vi "Message type that caused error.vi"(11 "ErrorHandler MsgPack in":refnum<class "ErrorHandler MsgPack.lvclass">) -> (2 "Error in response to message type":T1, 3 "ErrorHandler MsgPack out":refnum<class "ErrorHandler MsgPack.lvclass">)   [LabVIEW 2020, in "wamplv.lvlib" / "ErrorHandler MsgPack.lvclass"]
uses:
  ErrorHandler MsgPack.lvclass
  ErrorHandler MsgPack.lvclass/ErrorHandler MsgPack.ctl
  TypeDefs/WAMP Message Codes.ctl
  wamplv.lvlib
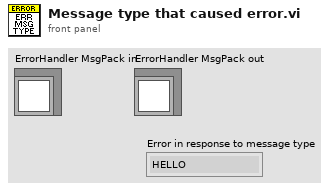
[diagram p1: front panel]
types:
  T1 = typedef "wamplv.lvlib/WAMP Message Codes.ctl" = enum8{"HELLO", "WELCOME", "CHALLENGE", "AUTHENTICATE", "ABORT", "GOODBYE", "ERROR", "PUBLISH", "PUBLISHED", "SUBSCRIBE", "SUBSCRIBED", "UNSUBSCRIBE", "UNSUBSCRIBED", "EVENT", "CALL", "RESULT", "REGISTER", "REGISTERED", "UNREGISTER", "UNREGISTERED", "INVOCATION", "YIELD"}
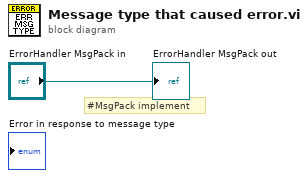
[diagram p0: block diagram]
diagram:
  # "#MsgPack implement"
  "ErrorHandler MsgPack out" <- "ErrorHandler MsgPack in"
